vi "ReadLidar.vi"(7 "error in (no error)":errorcluster, 10 "I2C Ref In":T1={"myRIO Reference"={"myRIO Model"=enum."Unknown", "myRIO Hardware Reference"={"Generic FPGA Reference"=refnum, "Allow multiple opens"=FALSE}}, "I2C Channels Enum"=enum."Not Connected", "I2C Configuration"={"I2C Transfer Rate"=enum."Fast mode (400 kbps)"}}) -> (0 "error out":errorcluster, 2 "Range (inches)":sgl)   [LabVIEW 2015]
uses:
  <vilib>/myRIO/Instrument Drivers/Onboard IO/I2C/typedefs/I2C Reference.ctl
  <vilib>/myRIO/Common/Instrument Driver Framework/Utilities/typedefs/myRIO Generic Hardware Reference.ctl
  <vilib>/myRIO/Common/Instrument Driver Framework/Utilities/typedefs/Hardware Version Enum.ctl
  <vilib>/myRIO/Common/Instrument Driver Framework/Utilities/typedefs/myRIO v1.0 Reference.ctl
  <vilib>/myRIO/Common/Instrument Driver Framework/Utilities/typedefs/Generic FPGA Reference.ctl
  <vilib>/myRIO/Common/Instrument Driver Framework/myRIO v1.0/I2C/typedefs/I2C Channels Enum.ctl
  <vilib>/myRIO/Instrument Drivers/Onboard IO/I2C/typedefs/I2C Configuration.ctl
  <vilib>/myRIO/Instrument Drivers/Onboard IO/I2C/typedefs/I2C Transfer Rate.ctl
  <vilib>/Utility/error.llb/Error Cluster From Error Code.vi
  <vilib>/myRIO/Common/Instrument Driver Framework/myRIO v1.0/I2C/vis/myRIO v1.0 Write I2C.vi
  <vilib>/myRIO/Common/Instrument Driver Framework/myRIO v1.0/I2C/vis/myRIO v1.0 Read I2C.vi
  <vilib>/myRIO/Instrument Drivers/Onboard IO/I2C/I2C.lvlib
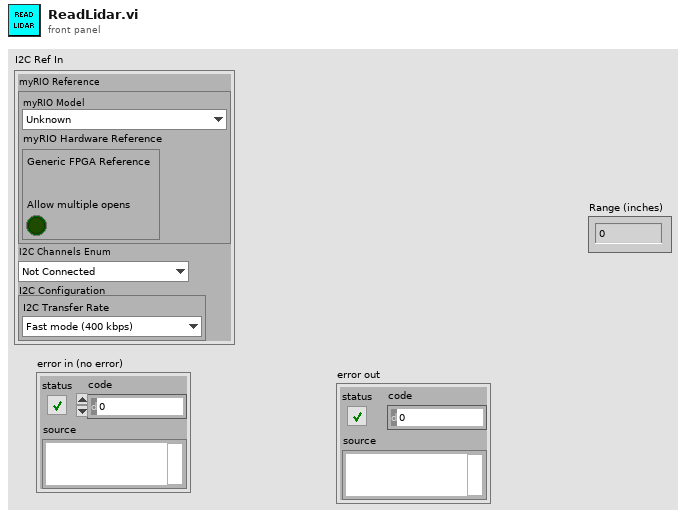
[diagram p1: front panel]
types:
  T1 = typedef "I2C.lvlib/I2C Reference.ctl" = cluster{"myRIO Reference":T2, "I2C Channels Enum":T6, "I2C Configuration":T7}
  T2 = typedef "myRIO Generic Hardware Reference.ctl" = cluster{"myRIO Model":T3, "myRIO Hardware Reference":T4}
  T3 = typedef "Hardware Version Enum.ctl" = enum16{"Unknown", "myRIO-1900", "myRIO-1950", "roboRIO"}
  T4 = typedef "myRIO v1.0 Reference.ctl" = cluster{"Generic FPGA Reference":T5, "Allow multiple opens":bool}
  T5 = typedef "Generic FPGA Reference.ctl" = refnum<k20>
  T6 = typedef "I2C Channels Enum.ctl" = enum16{"Not Connected", "A/I2C", "B/I2C", "I2C/I2C"}
  T7 = typedef "I2C.lvlib/I2C Configuration.ctl" = cluster{"I2C Transfer Rate":T8}
  T8 = typedef "I2C.lvlib/I2C Transfer Rate.ctl" = enum16{"Standard mode (100 kbps)", "Fast mode (400 kbps)"}
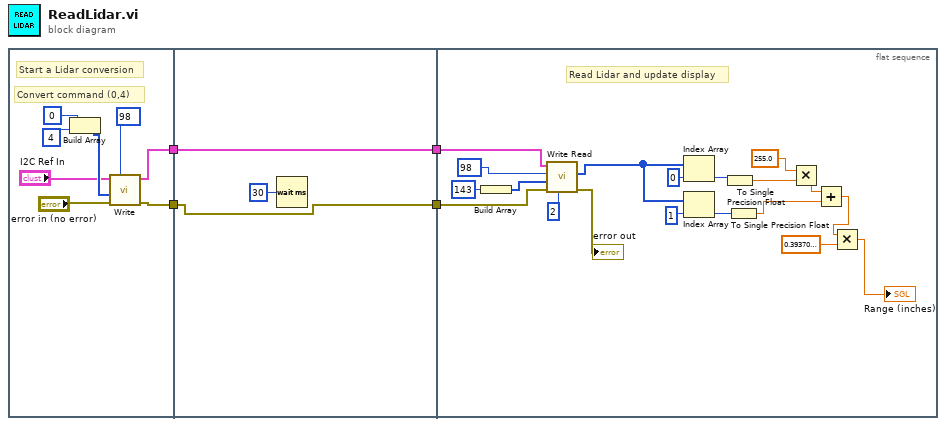
[diagram p0: block diagram]
diagram:
  n1 = flat-sequence {
    tunnel: [w7] -> w4
    tunnel: [w6] -> w2
    tunnel: w4 -> [w14]
    tunnel: [w14] -> w3
    tunnel: w2 -> [w13]
    tunnel: [w13] -> w1
    tunnel: w3 -> [w17]
    tunnel: w1 -> [w16]
    frame #0 {
      # "Start a Lidar conversion"
      # "Convert command (0,4)"
      n2 = Build Array(u8 0 ("Slave Address (7-bit)"), u8 4 ("Slave Address (7-bit)")) -> (w9:u8[])
      n3 = call <vilib>:"Write.vi"("error in (no error)"="error in (no error)", "Bytes to Write"=w9, "Slave Address (7-bit)"=u8 98, "I2C Ref In"="I2C Ref In") -> ("error out"=w6:errorcluster, "I2C Ref Out"=w7:T1)  [unwired: 6 in]
    }
    frame #1 {
      n4 = Wait (ms)(milliseconds to wait=u32 30) -> ()  [unwired: 1 out]
    }
    frame #2 {
      # "Read Lidar and update display"
      n5 = Build Array(u8 143 ("Slave Address (7-bit)")) -> (w19:u8[])
      n6 = call <vilib>:"Write Read.vi"("Byte Count"=u32 2, "error in (no error)"=w16, "Bytes to Write"=w19, "Slave Address (7-bit)"=u8 98, "I2C Ref In"=w17) -> ("error out"=→"error out":errorcluster, "Bytes Read"=w26:u8[])  [unwired: 3 in, 1 out]
      n7 = Index Array(array=w26, index=0) -> (element=w25:u8)
      n8 = Index Array(array=w26, index=1) -> (element=w23:u8)
      n9 = To Single Precision Float(number=w25) -> (single precision float=w24:sgl)
      n10 = To Single Precision Float(number=w23) -> (single precision float=w22:sgl)
      n11 = Multiply(x=sgl 255.0 ("y"), y=w24) -> (x*y=w30:sgl)
      n12 = Add(x=w30, y=w22) -> (x+y=w31:sgl)
      n13 = Multiply(x=w31, y=sgl 0.3937) -> (x*y=→"Range (inches)":sgl)
    }
  }
